vi "filter_02.vi"(1 "SignalIn":waveform(i16)) -> (0 "SignalOut":waveform(i16))   [LabVIEW 2010]
uses:
  <vilib>/Analysis/3filter.llb/Bessel Filter (DBL).vi
  <vilib>/Analysis/NI_AALBase.lvlib
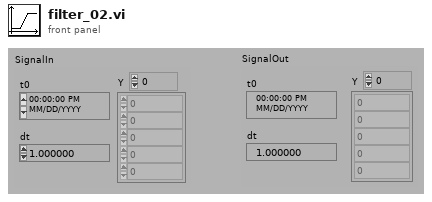
[diagram p1: front panel]
types:
  T1 = enum32{"Lowpass", "Highpass", "Bandpass", "Bandstop"}
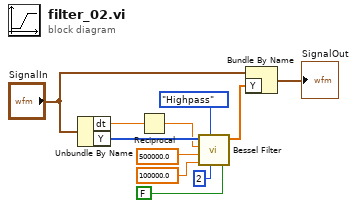
[diagram p0: block diagram]
diagram:
  n1 = Unbundle By Name("SignalIn") -> ("dt"=w3:dbl, "Y"=w11:i16[])
  n2 = Reciprocal(x=w3) -> (1/x=w8:dbl)
  n3 = call-poly <vilib>:"Bessel Filter.vi"("init/cont (init:F)"=FALSE, "order"=2, "filter type"=T1."Highpass", "low cutoff freq: fl"=100000.0 ("stop freq"), "high cutoff freq: fh"=500000.0 ("high freq"), "sampling freq: fs"=w8, "X"=w11) -> ("Filtered X"=w5:dbl[])  [unwired: 1 in, 1 out]
  n4 = Bundle By Name(cluster="SignalIn", "Y"=w5) -> (→"SignalOut":waveform(i16))
